vi "main.vi"() -> ()   [LabVIEW 2024]
uses:
  Module1/Module 1.lvlib
  Module2/Module 2.lvlib
  Module 1 Cases.ctl
  Module 2 Cases.ctl
  <extravilib>/ChannelInstances/Event Messenger-t'Channel Messages.lvlib-Message Cluster.ctl'.lvlib
  71319344-41ff-4242-989e-c571bc358f37.vi
  Module Main Cases.ctl
  a7e4e8bb-eedc-4424-851a-ea56d93da92e.vi
  6921bc99-b2d4-40c6-9ade-ed48eb012b80.vi
  9a93f236-a99b-42dd-b4c6-054a9b440e74.vi
  Common-LabVIEW-Helpers/Source/Common Helpers.lvlib
panel:
  in  "Show Module2":bool
  in  "Show Module1":bool
  in  "Process Stop Button":bool
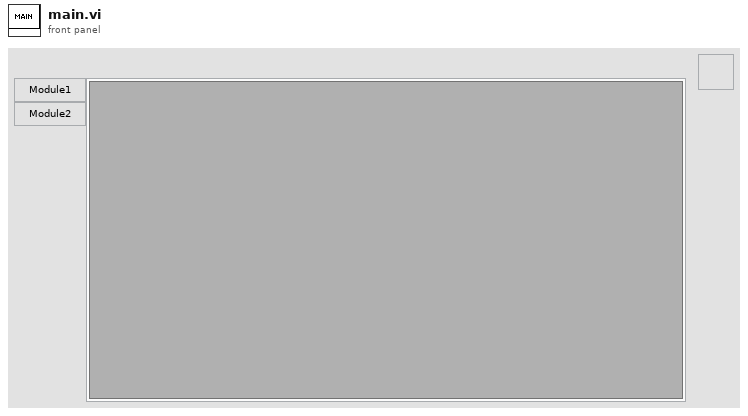
[diagram p1: front panel]
types:
  T1 = typedef "Module 2 Cases.ctl" = enum16{"Kill", "Stop", "Start", "Log"}
  T2 = typedef "Module 1 Cases.ctl" = enum16{"Kill", "Log", "Stop", "Init", "Sum"}
  T3 = typedef "Module Main Cases.ctl" = enum16{"Error", "Log"}
  T4 = typedef "Channel Messages.lvlib/Message Cluster.ctl" = cluster{"Cmd":string, "Data":variant}
  T5 = typedef "Event Messenger-t'Channel Messages.lvlib-Message Cluster.ctl'.lvlib/))Channel.ctl" = refnum<queue>
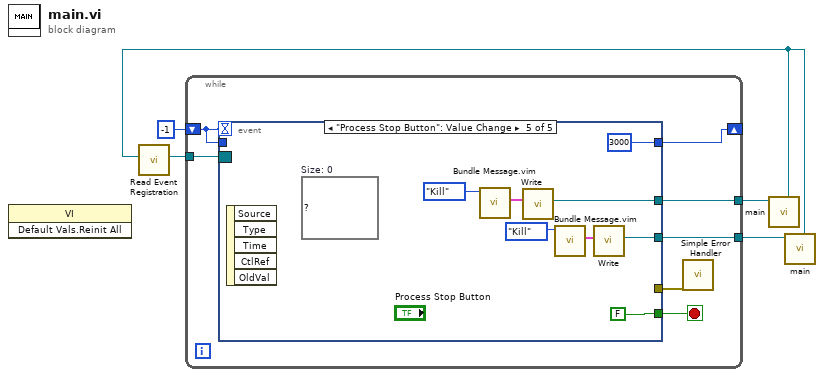
[diagram p0: block diagram]
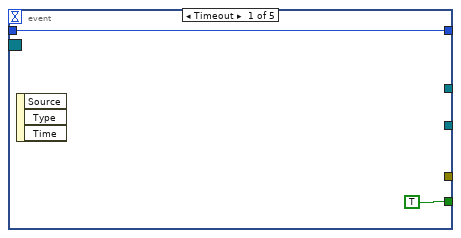
[diagram p2: hidden frame]
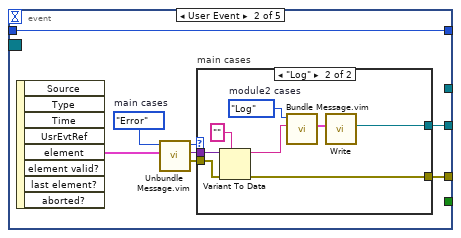
[diagram p3: hidden frame]
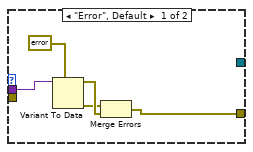
[diagram p4: hidden frame]
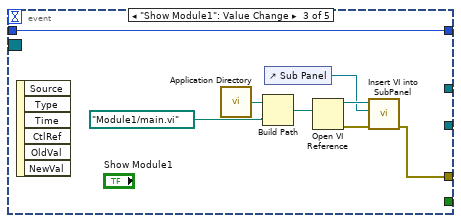
[diagram p5: hidden frame]
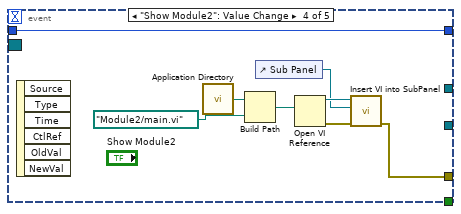
[diagram p6: hidden frame]
diagram:
  n1 = invoke class="VI" method="Default Vals.Reinit All"() -> ()  [unwired: 3 in, 3 out]
  n2 = call <extravilib>:"Read Event Registration.vi"("channel"=w2) -> ("event registration refnum"=w4:refnum<event-registration>)  [unwired: 10 in]
  n3 = while {
    tunnel: [w10] -> w3
    tunnel: [w11] -> w5
    tunnel: w4 -> [w8]
    shift-right: [w7] -> _
    shift-left: -1 -> [w6]
    stop <- w12 stop-if-true
    n4 = event shown="[4] \"Process Stop Button\": Value Change" {
      selector: w8 -> [_ _ _ _ _]
      dyn-events: _ -> [_ _ _ _ _]
      timeout: w6 -> [_ _ _ _ _]
      tunnel: [TRUE _ _ _ FALSE] -> w12
      tunnel: [_ _ _ _ w59] -> w11
      tunnel: [_ w18 _ _ w58] -> w10
      tunnel: [_ w19 w36 w44 _] -> w9
      tunnel: [w14 w17 w43 w51 3000] -> w7
      tunnel: w6 -> [w14 w17 w43 w51 _]
      event Timeout {
        n5 = event-data() -> ()  [unwired: 1 in, 3 out]
      }
      event User Event {
        w22 = Module_Main_Cases."Error"  # main cases
        n6 = event-data() -> ("element"=w15:T4)  [unwired: 1 in, 7 out]
        n7 = call "Unbundle Message.vim"("message"=w15, "case type"=w22) -> ("error out"=w16:errorcluster, "data"=w20:variant, "case"=w21:T3)  [unwired: 7 in]
        n8 = case "main cases" shown="\"Log\"" w21 {
          tunnel: w20 -> [w27 w35]
          tunnel: [w24 w33] -> w19
          tunnel: [_ w29] -> w18
          tunnel: w16 -> [_ w28]
          frame "Error", Default {
            n9 = Variant To Data(type=errorcluster {"status"=FALSE, "code"=0, "source"=""} ("error constant"), Variant=w27) -> (data=w25:errorcluster, error out=w23:errorcluster)  [unwired: 1 in]
            n10 = Merge Errors(w23, w25) -> (w24:errorcluster)
          }
          frame "Log" {
            w32 = Module_2_Cases."Log"  # module2 cases
            n11 = Variant To Data(error in=w28, type="", Variant=w35) -> (data=w31:string, error out=w33:errorcluster)
            n12 = call "Bundle Message.vim"("data"=w31, "case"=w32) -> ("message"=w30:T4)  [unwired: 9 in]
            n13 = call <extravilib>:"Write.vi"("element"=w30) -> ("channel"=w29:T5)  [unwired: 9 in, 1 out]
          }
        }
      }
      event "Show Module1": Value Change {
        n14 = event-data() -> ()  [unwired: 1 in, 6 out]
        n15 = call <vilib>:"Application Directory.vi"() -> ("Application Directory"=w42:path)
        n16 = Build Path(base path=w42, name or relative path=path "Module1/main.vi") -> (appended path=w41:path)
        n17 = control-ref of="Sub Panel"() -> (w38:refnum<vi>)
        n18 = Open VI Reference(vi path=w41) -> (vi reference=w40:refnum<vi>, error out=w39:errorcluster)  [unwired: 5 in]
        n19 = call "Insert VI into SubPanel.vi"("error in"=w39, "SubPnl Ref"=w38, "VI Ref"=w40) -> ("error out"=w36:errorcluster)  [unwired: 7 in, 1 out]
      }
      event "Show Module2": Value Change {
        n20 = event-data() -> ()  [unwired: 1 in, 6 out]
        n21 = call <vilib>:"Application Directory.vi"() -> ("Application Directory"=w50:path)
        n22 = Build Path(base path=w50, name or relative path=path "Module2/main.vi") -> (appended path=w49:path)
        n23 = control-ref of="Sub Panel"() -> (w46:refnum<vi>)
        n24 = Open VI Reference(vi path=w49) -> (vi reference=w48:refnum<vi>, error out=w45:errorcluster)  [unwired: 5 in]
        n25 = call "Insert VI into SubPanel.vi"("error in"=w45, "SubPnl Ref"=w46, "VI Ref"=w48) -> ("error out"=w44:errorcluster)  [unwired: 7 in, 1 out]
      }
      event "Process Stop Button": Value Change {
        (unwired) map{T2, i32} {}  # Size: 0
        n26 = event-data() -> ()  [unwired: 1 in, 5 out]
        n27 = call "Bundle Message.vim"("case"=Module_1_Cases."Kill" ("Case")) -> ("message"=w55:T4)  [unwired: 10 in]
        n28 = call <extravilib>:"Write.vi"("element"=w55) -> ("channel"=w59:T5)  [unwired: 9 in, 1 out]
        n29 = call "Bundle Message.vim"("case"=Module_2_Cases."Kill" ("Case")) -> ("message"=w53:T4)  [unwired: 10 in]
        n30 = call <extravilib>:"Write.vi"("element"=w53) -> ("channel"=w58:T5)  [unwired: 9 in, 1 out]
      }
    }
    n31 = call <vilib>:"Simple Error Handler.vi"("error in (no error)"=w9) -> ()  [unwired: 4 in, 5 out]
  }
  n32 = call "main.vi"("Message Input"=w5) -> ("Message Output"=w2:T5)  [unwired: 10 in]
  n33 = call "main.vi"("Message Output"=w2, "Message Input"=w3) -> ()  [unwired: 10 in]
